vi "S3-SenseBall.vi"(0 "Ball S3 Process":bool, 2 "Sense Ball":bool, 3 "Trigger Shooter":bool) -> (7 "Ball Counter":dbl, 8 "Trigger Shooter Output":bool, 9 "Ball S3 Process Output":bool, 10 "Conveyer Output":dbl)   [LabVIEW 2011]
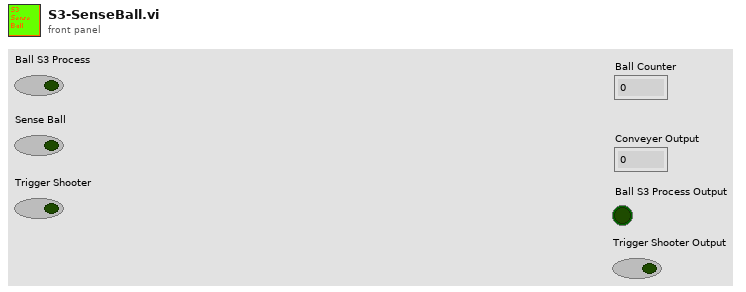
[diagram p1: front panel]
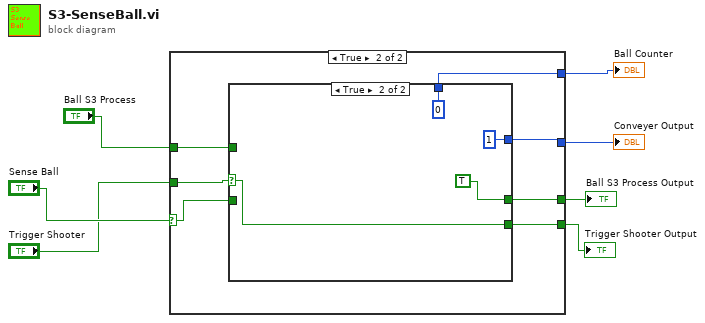
[diagram p0: block diagram]
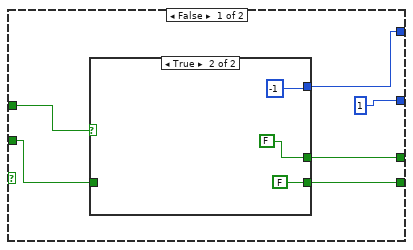
[diagram p2: hidden frame]
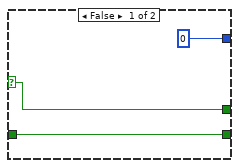
[diagram p3: hidden frame]
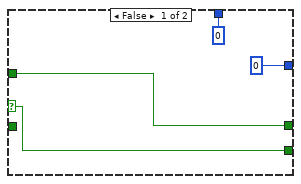
[diagram p4: hidden frame]
diagram:
  n1 = case shown="True" "Sense Ball" {
    selector: "Sense Ball" -> [_ w24]
    tunnel: [1 w25] -> w6
    tunnel: "Trigger Shooter" -> [w9 w26]
    tunnel: [w10 w23] -> w4
    tunnel: "Ball S3 Process" -> [w12 w20]
    tunnel: [w11 w22] -> w2
    tunnel: [w8 w21] -> w1
    frame False {
      n2 = case shown="True" w12 {
        selector: w12 -> [w14 _]
        tunnel: [w15 FALSE] -> w11
        tunnel: [0 -1] -> w10
        tunnel: w9 -> [w15 _]
        tunnel: [w14 FALSE] -> w8
        frame False {
        }
        frame True {
        }
      }
    }
    frame True {
      n3 = case shown="True" w26 {
        selector: w26 -> [w28 w32]
        tunnel: [0 1] -> w25
        tunnel: w24 -> [_ _]
        tunnel: [0 0] -> w23
        tunnel: [w28 w32] -> w22
        tunnel: [w27 TRUE] -> w21
        tunnel: w20 -> [w27 _]
        frame False {
        }
        frame True {
        }
      }
    }
  }
  "Conveyer Output" <- w6
  "Ball Counter" <- w4
  "Ball S3 Process Output" <- w1
  "Trigger Shooter Output" <- w2
